vi "dlltest.vi"() -> ()   [LabVIEW 2017]
uses:
  D:/Documents/Visual Studio 2015/Projects/labsqrt/x64/Release/labsqrt.dll
panel:
  out "arg1":dbl
  out "arg2":dbl
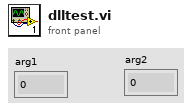
[diagram p1: front panel]
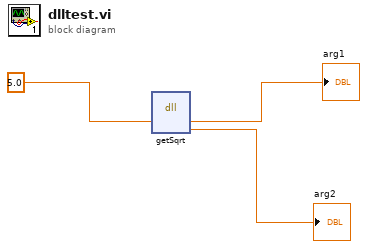
[diagram p0: block diagram]
diagram:
  n1 = dll-call lib="D:/Documents/Visual Studio 2015/Projects/labsqrt/x64/Release/labsqrt.dll" fn="getSqrt"("arg1"=5.0) -> ("arg1"=→"arg1":dbl, "arg2"=→"arg2":dbl)  [unwired: 5 in, 2 out]
